vi "Initialize Sine.vi"(7 "Sample Count":dbl, 8 "error in (no error)":errorcluster, 9 "Frequency":dbl, 10 "Amplitude":dbl, 11 "Sine Stimulus in":refnum<class "Sine Stimulus.lvclass">) -> (0 "error out":errorcluster, 3 "Sine Stimulus out":refnum<class "Sine Stimulus.lvclass">)   [LabVIEW 2015, in "Sine Stimulus.lvclass"]
uses:
  Sine Stimulus.lvclass
  Sine Stimulus.lvclass/Sine Stimulus.ctl
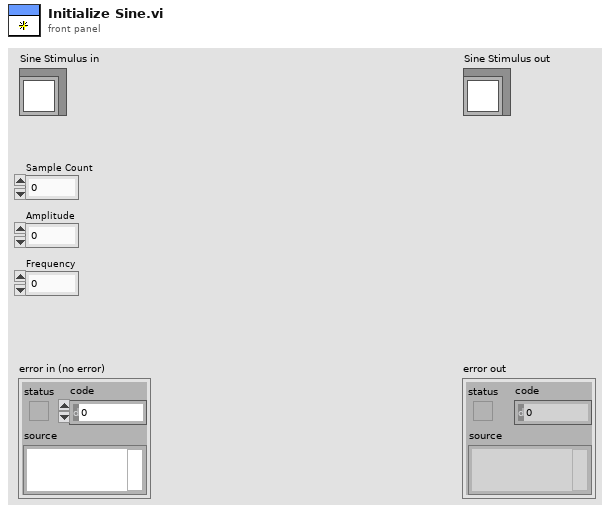
[diagram p1: front panel]
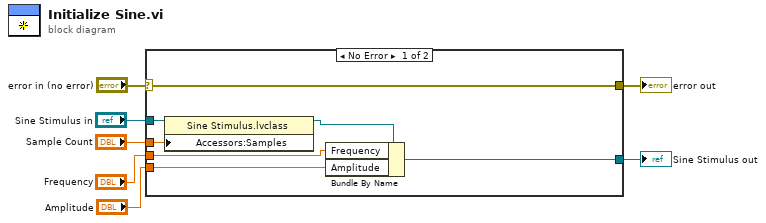
[diagram p0: block diagram]
diagram:
  n1 = case shown="No Error" "error in (no error)" {
    selector: "error in (no error)" -> [w14 w16]
    tunnel: [w14 w16] -> w6
    tunnel: [w10 w15] -> w4
    tunnel: "Sine Stimulus in" -> [w13 w15]
    tunnel: "Sample Count" -> [w12 _]
    tunnel: "Frequency" -> [w9 _]
    tunnel: "Amplitude" -> [w8 _]
    frame No Error {
      n2 = property class="Sine Stimulus.lvclass"(reference=w13, "Accessors:Samples"=w12) -> (reference out=w11:refnum<class "Sine Stimulus.lvclass">)  [unwired: 1 in, 1 out]
      n3 = Bundle By Name(cluster=w11, "Frequency"=w9, "Amplitude"=w8) -> (w10:refnum<class "Sine Stimulus.lvclass">)
    }
    frame Error {
    }
  }
  "error out" <- w6
  "Sine Stimulus out" <- w4
